vi "2D_Array_DualSort_SubSortReversed.vi"(0 "RawArray":string[][](array[string]), 7 "PrimarySortColumn":i32, 11 "SubSortColumn":i32) -> (4 "SortedArray":string[][](array[string]), 15 "DesiredParameters":string)   [LabVIEW 2013]
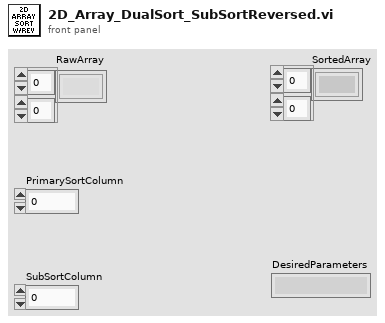
[diagram p1: front panel]
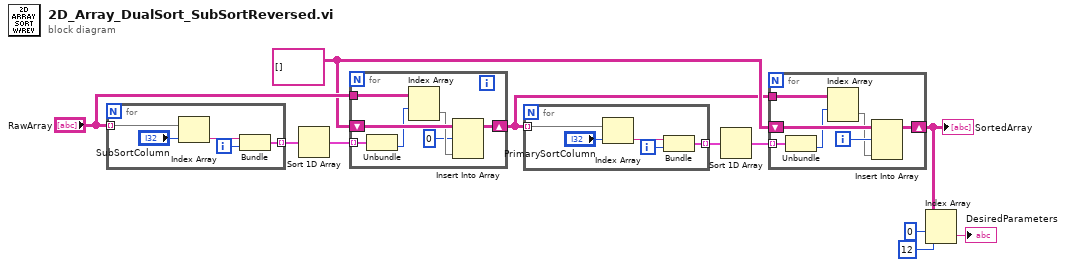
[diagram p0: block diagram]
diagram:
  w6 = string[][] []
  n1 = for {
    tunnel: "RawArray" -> [w15] mode=indexing
    tunnel: [w16] -> w11 mode=indexing
    i -> [w12]
    n2 = Index Array(array=w15, index="SubSortColumn") -> (element=w14:string)
    n3 = Bundle("String"=w14, w12) -> (w16:cluster{"String":string, i32})  [unwired: 1 in]
  }
  n4 = Sort 1D Array(array=w11) -> (sorted array=w9:cluster{"String":string, i32}[])
  n5 = for {
    tunnel: "RawArray" -> [w21]
    shift-right: [w22] -> w5
    shift-left: w6 -> [w23]
    tunnel: w9 -> [w20] mode=indexing
    n6 = Unbundle(w20) -> (w19:i32)  [unwired: 1 out]
    n7 = Index Array(array=w21, index (row)=w19) -> (element=w18:string[])  [unwired: 1 in]
    n8 = Insert Into Array(array=w23, index (row)=0, new element=w18) -> (w22:string[][])  [unwired: 1 in]
  }
  n9 = for {
    tunnel: w5 -> [w27] mode=indexing
    tunnel: [w28] -> w8 mode=indexing
    i -> [w25]
    n10 = Index Array(array=w27, index="PrimarySortColumn") -> (element=w26:string)
    n11 = Bundle(w26, w25) -> (w28:cluster{string, i32})  [unwired: 1 in]
  }
  n12 = Sort 1D Array(array=w8) -> (sorted array=w7:cluster{string, i32}[])
  n13 = for {
    tunnel: w5 -> [w32]
    shift-right: [w34] -> w4
    shift-left: w6 -> [w35]
    tunnel: w7 -> [w31] mode=indexing
    i -> [w33]
    n14 = Unbundle(w31) -> (w30:i32)  [unwired: 1 out]
    n15 = Index Array(array=w32, index (row)=w30) -> (element=w29:string[])  [unwired: 1 in]
    n16 = Insert Into Array(array=w35, index (row)=w33, new element=w29) -> (w34:string[][])  [unwired: 1 in]
  }
  "SortedArray" <- w4
  n17 = Index Array(array=w4, index (row)=0, index (col)=12 ("disabled index (col)")) -> (element=→"DesiredParameters":string)
